vi "运维调试_五参数.vi"(11 "编号":string) -> ()   [LabVIEW 2022 SP3, in "斯坦道多参数.lvlib"]
uses:
  <vilib>/Utility/miscctls.llb/LVPointTypeDef.ctl
  <vilib>/Plasmionique/MB Master/MB_Master/MB_Master.lvclass
  <vilib>/ptbypt/NI_PtbyPt.lvlib
  <vilib>/Utility/config.llb/NI_LVConfig.lvlib
  <userlib>/_OpenG.lib/variantconfig/variantconfig.llb/openg_variant_configuration_file.lvlib
panel:
  in  "Serial Config":T1={"baud rate (bps)"=9600, "stop bits"=10, "parity"=0, "flow control"=0, "timeout"=2000, "retries"=1} {"stop bits" items=["1.0"=10, "1.5"=15, "2.0"=20]; "parity" items=["None", "Odd", "Even", "Mark", "Space"]; "flow control" items=["None", "XON/XOFF", "RTS/CTS", "XON/XOFF & RTS/CTS", "DTR/DSR", "XON/XOFF & DTR/DSR"]}
  in  "探头设置":bool
  in  "量程设置":bool
  out "显示框":T2={"显示控件"={"标题背景颜色"=3381759, "监测值背景颜色"=16777226, "监测参数"="", "状态1"="", "状态2"="", "数据标识"=""}, "显示控件 2"={"标题背景颜色"=3381759, "监测值背景颜色"=16777226, "监测参数"="", "状态1"="", "状态2"="", "数据标识"=""}, "显示控件 3"={"标题背景颜色"=3381759, "监测值背景颜色"=16777226, "监测参数"="", "状态1"="", "状态2"="", "数据标识"=""}, "显示控件 4"={"标题背景颜色"=3381759, "监测值背景颜色"=16777226, "监测参数"="", "状态1"="", "状态2"="", "数据标识"=""}, "显示控件 5"={"标题背景颜色"=3381759, "监测值背景颜色"=16777226, "监测参数"="", "状态1"="", "状态2"="", "数据标识"=""}, "显示控件 6"={"标题背景颜色"=3381759, "监测值背景颜色"=16777226, "监测参数"="", "状态1"="", "状态2"="", "数据标识"=""}, "显示控件 7"={"标题背景颜色"=3381759, "监测值背景颜色"=16777226, "监测参数"="", "状态1"="", "状态2"="", "数据标识"=""}, "显示控件 8"={"标题背景颜色"=3381759, "监测值背景颜色"=16777226, "监测参数"="", "状态1"="", "状态2"="", "数据标识"=""}, "显示控件 9"={"标题背景颜色"=3381759, "监测值背景颜色"=16777226, "监测参数"="", "状态1"="", "状态2"="", "数据标识"=""}, "显示控件 10"={"标题背景颜色"=3381759, "监测值背景颜色"=16777226, "监测参数"="", "状态1"="", "状态2"="", "数据标识"=""}}
  in  "传感器系列号":bool
  in  "水样保存组数":dbl caption="水样保存组数:"
  in  "水样稳定时间":dbl caption="水样稳定时间:"
  out "模块版本号":string
  out "权限等级":string
  in  "打开modbus":bool
  out "选项卡控件":enum32{"选项卡 1", "选项卡 2"}(tab)
  in  "VISA资源名称":refnum<visa-resource-name> caption="串口"
  in  "IP":string="localhost" caption="IP:"
  in  "Port":u16=502 caption="Port:"
  in  "自动断线重连":bool=TRUE
  in  "连接方式":u16(ring) items=["Modbus RTU", "Modbus TCP"]
  in  "密码锁":bool
  in  "设置页返回":bool
  in  "周期设置":bool
  out "当前串口":string
  out "运行状态":enum16{"空闲", "水样测试", "标样核查"}(ring)
  in  "停止":bool
  in  "标样核查":bool
  in  "水样测试":bool
  in  "设置":bool
  in  "探头校正返回":bool
  in  "探头校正":bool
  # "请设置仪器连接方式"
  # "组"
  # "min"
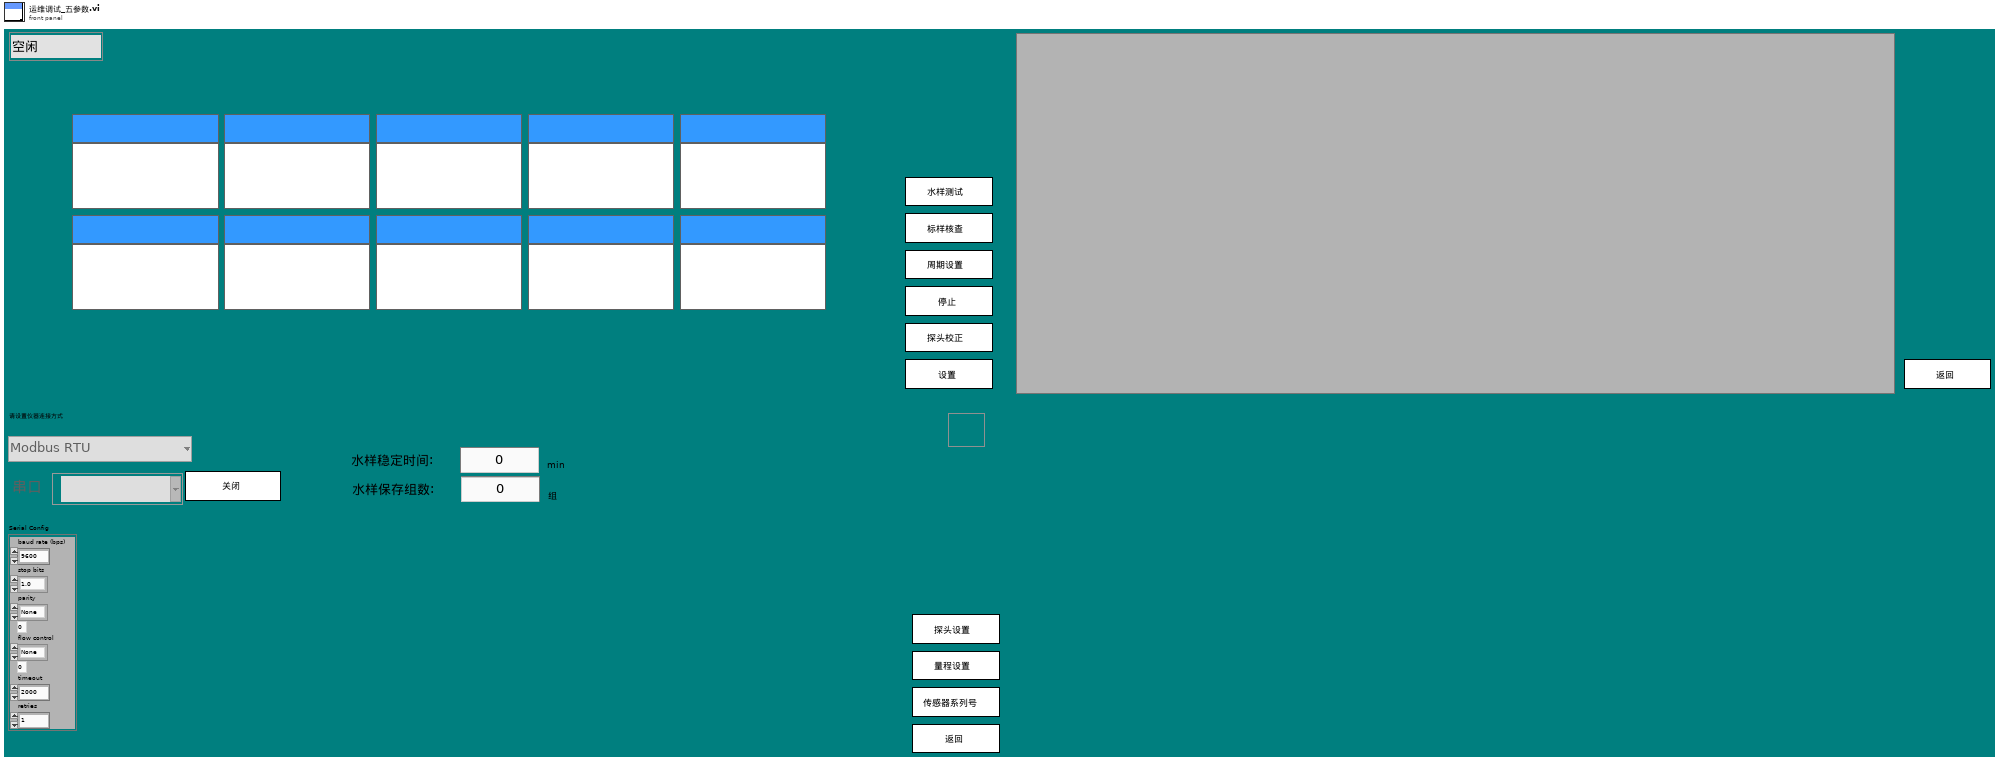
[diagram p1: front panel]
types:
  T1 = cluster{"baud rate (bps)":u32, "stop bits":u16, "parity":u16, "flow control":u16, "timeout":u32, "retries":i32}
  T2 = typedef "斯坦道多参数.lvlib/多状态显示框.ctl" = cluster{"显示控件":T3, "显示控件 2":T3, "显示控件 3":T3, "显示控件 4":T3, "显示控件 5":T3, "显示控件 6":T3, "显示控件 7":T3, "显示控件 8":T3, "显示控件 9":T3, "显示控件 10":T3}
  T3 = typedef "斯坦道多参数.lvlib/显示控件.ctl" = cluster{"标题背景颜色":u32, "监测值背景颜色":u32, "监测参数":string, "状态1":string, "状态2":string, "数据标识":string}
  T4 = typedef "斯坦道多参数.lvlib/数据流类型.ctl" = cluster{"cmd":enum16{"水样测试", "标样核查", "校准状态同步", "停止"}, "data":variant}
  T5 = typedef "LVPointTypeDef.ctl" = cluster{"Horizontal":i16, "Vertical":i16}
  T6 = enum8{"Enabled", "Disabled", "Disabled and Grayed Out"}
  T7 = cluster{"标签":string, "检测值1":cluster{"检测值":dbl, "单位":string, "启用":bool}, "检测值2":cluster{"检测值":dbl, "单位":string, "启用":bool}, "数据标识":string}[]
  T8 = cluster{"标签":string, "检测值1":cluster{"检测值":dbl, "单位":string, "启用":bool}, "检测值2":cluster{"检测值":dbl, "单位":string, "启用":bool}, "数据标识":string}
  T9 = cluster{"CH":u16, "监测值":dbl, "信号值":sgl, "数据标识":string}
  T10 = cluster{"温度测量值":sgl, "测量值":sgl, "温度偏移修正值":sgl, "信号值":sgl, "数据标识":string}
  T11 = cluster{"温度测量值":sgl, "DO%":sgl, "DOmg/L":sgl, "温度偏移修正值":sgl, "数据标识mg/L":string, "数据标识%":string}
  T12 = cluster{"周期设置类型":enum16{"定点启动", "间隔启动"}, "定时功能启用":bool, "定时间隔":u32, "24H周期设置":bool[], "延迟启动时间":u32}
  T13 = typedef "LVDateTimeRec.ctl" = cluster{"秒数的小数部分":dbl, "秒":i32, "分":i32, "时":i32, "日":i32, "月":i32, "年":i32, "天数（周）":i32, "天数（年）":i32, "DST":i32}
  T14 = cluster{"运行模式":enum16{"维护模式", "常规模式", "应急模式", "质控模式"}, "24H周期设置":bool[]}
  T15 = cluster{"Major":u16, "Minor":u16, "Fix":u16, "Build":u16}
  T16 = typedef "NI_LVConfig.lvlib/Config Data RefNum.ctl" = refnum<k1>
  T17 = enum32{"Bad", "Idle", "Run top level", "Running"}
  T18 = cluster{"ph":bool, "DO":bool, "Cond":bool, "Turb":bool, "叶绿素a":bool, "藻密度":bool, "ORP":bool, "cod":bool, "DO2":bool, "氯化物":bool, "氨氮":bool, "水中油":bool, "悬浮物":bool, "余氯":bool}
  T19 = cluster{"水温 (℃)":cluster{"量程下限":dbl, "量程上限":dbl}, "DO (mg/L)":cluster{"量程下限":dbl, "量程上限":dbl}, "DO (%)":cluster{"量程下限":dbl, "量程上限":dbl}, "pH":cluster{"量程下限":dbl, "量程上限":dbl}, "电导率 (μS/cm)":cluster{"量程下限":dbl, "量程上限":dbl}, "盐度":cluster{"量程下限":dbl, "量程上限":dbl}, "浊度 (NTU)":cluster{"量程下限":dbl, "量程上限":dbl}, "叶绿素a (μg/L)":cluster{"量程下限":dbl, "量程上限":dbl}, "藻密度 (cells/mL)":cluster{"量程下限":dbl, "量程上限":dbl}, "ORP (mV)":cluster{"量程下限":dbl, "量程上限":dbl}, "氯化物（mg/L）":cluster{"量程下限":dbl, "量程上限":dbl}, "COD":cluster{"量程下限":dbl, "量程上限":dbl}, "氨氮":cluster{"量程下限":dbl, "量程上限":dbl}, "水中油":cluster{"量程下限":dbl, "量程上限":dbl}, "悬浮物":cluster{"量程下限":dbl, "量程上限":dbl}, "余氯":cluster{"量程下限":dbl, "量程上限":dbl}}
  T20 = cluster{"周期设置类型":enum16{"定点启动", "间隔启动"}, "定时功能启用":bool, "定时间隔":u32, "24H周期设置":bool[], "延时启动时间":u32}
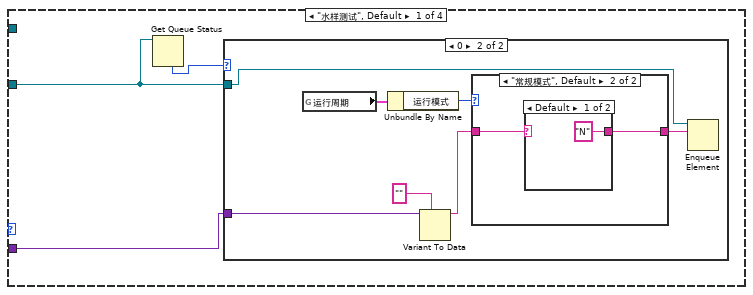
[diagram p2: hidden frame]
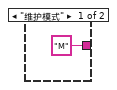
[diagram p4: hidden frame]
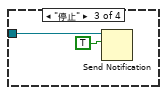
[diagram p7: hidden frame]
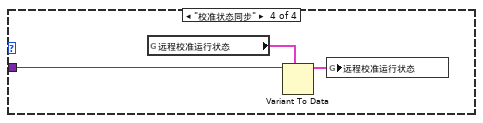
[diagram p8: hidden frame]
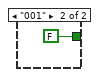
[diagram p9: hidden frame]
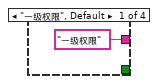
[diagram p17: hidden frame]
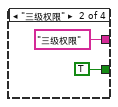
[diagram p18: hidden frame]
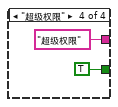
[diagram p19: hidden frame]
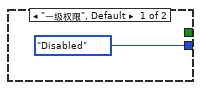
[diagram p20: hidden frame]
diagram:
  n1 = control-ref of="本VI"() -> (w22:refnum<vi>)
  n2 = while {
    stop <- FALSE stop-if-true
    n3 = global read "多参数全局变量.vi" "多参数运行状态"() -> (→"运行状态":u16)
    n4 = Wait (ms)(milliseconds to wait=u32 1000 ("等待时间（毫秒）")) -> ()  [unwired: 1 out]
  }
  n5 = call "程序默认配置.vi"() -> ()  [unwired: 11 in, 1 out]
  n6 = while {
    stop <- FALSE stop-if-true
    # "配置"
    n7 = global read "断电保存变量.vi" "Port"() -> (w55:u16)
    n8 = global read "断电保存变量.vi" "IP"() -> (w56:string)
    n9 = global read "断电保存变量.vi" "连接方式"() -> (w49:u16)
    "选项卡控件" <- w49
    n10 = global read "多参数全局变量.vi" "MB session in"() -> (w64:refnum<class "MB_Master.lvclass">)
    n11 = Wait (ms)(milliseconds to wait=u32 500 ("等待时间（毫秒）")) -> ()  [unwired: 1 out]
    n12 = global read "断电保存变量.vi" "VISA资源名称"() -> (w52:refnum<visa-resource-name>)
    n13 = global read "断电保存变量.vi" "Serial Config"() -> (w40:T1)
    n14 = global read "断电保存变量.vi" "水样稳定时间"() -> (w43:dbl)
    n15 = global read "断电保存变量.vi" "水样测试组数"() -> (w41:dbl)
    n16 = global read "断电保存变量.vi" "自动断线重连"() -> (w44:bool)
    n17 = local write "IP"(w56) -> ()
    n18 = local write "Port"(w55) -> ()
    n19 = global read "断电保存变量.vi" "连接方式"() -> (w53:u16)
    n20 = local write "连接方式"(w49) -> ()
    n21 = local write "Serial Config"(w40) -> ()
    n22 = local write "水样稳定时间"(w43) -> ()
    n23 = global read "多参数全局变量.vi" "MB session in"() -> (w67:refnum<class "MB_Master.lvclass">)
    n24 = local write "水样保存组数"(w41) -> ()
    n25 = local write "自动断线重连"(w44) -> ()
    n26 = local write "VISA资源名称"(w52) -> ()
    n27 = case shown="1" w53 {
      tunnel: w52 -> [w69 _]
      tunnel: [w69 w70] -> w51
      frame 0, Default {
      }
      frame 1 {
        n28 = global read "断电保存变量.vi" "Port"() -> (w71:u16)
        n29 = global read "断电保存变量.vi" "IP"() -> (w73:string)
        n30 = Format Into String(format string=":%d" ("格式字符串"), initial string=w73, w71) -> (resulting string=w70:string)  [unwired: 1 in, 1 out]
      }
    }
    "当前串口" <- w51
    n31 = property class="MB_Master"(reference=w64) -> ("Properties:Session Valid"=w48:bool)  [unwired: 1 in, 2 out]
    n32 = local read "密码锁"() -> (w60:bool)
    n33 = property class="MB_Master"(reference=w67) -> ("Properties:Session Valid"=w66:bool)  [unwired: 1 in, 2 out]
    n34 = Select(t=T6."Enabled" ("f"), s=w60, f=T6."Disabled") -> (s? t:f=w58:T6)
    n35 = Not(x=w48) -> (.not. x?=w50:bool)
    n36 = Select(t="关闭" ("布尔文本.文本"), s=w48, f="打开" ("布尔文本.文本")) -> (s? t:f=w61:string)
    n37 = Select(t=u32 16777216, s=w48, f=u32 16722483) -> (s? t:f=w45:u32)
    n38 = property on="当前串口" class="Str"("Blinking"=w50, "Text.BG Color"=w45) -> ()  [unwired: 2 in, 2 out]
    n39 = Select(t=T6."Disabled and Grayed Out" ("禁用"), s=w66, f=w58) -> (s? t:f=w54:T6)
    n40 = property on="IP" class="Str"("DisabledEnum"=w54) -> ()  [unwired: 2 in, 2 out]
    n41 = property on="Port" class="DigNum (strict)"("DisabledEnum"=w54) -> ()  [unwired: 2 in, 2 out]
    n42 = property on="VISA资源名称" class="VISAName"("DisabledEnum"=w54) -> ()  [unwired: 2 in, 2 out]
    n43 = property on="连接方式" class="Ring (strict)"("DisabledEnum"=w54) -> ()  [unwired: 2 in, 2 out]
    n44 = property on="打开modbus" class="Bool"("BoolText.Text"=w61) -> ()  [unwired: 2 in, 2 out]
  }
  n45 = call "taskqueue ref.vi"() -> ("队列输出"=w5:refnum<queue>)  [unwired: 10 in, 1 out]
  n46 = while {
    stop <- FALSE stop-if-true
    # "显示处理"
    n47 = global read "断电保存变量.vi" "Temp"() -> (w121:bool)
    n48 = Wait (ms)(milliseconds to wait=u32 1000 ("等待时间（毫秒）")) -> ()  [unwired: 1 out]
    n49 = case shown="True" w121 {
      tunnel: [w401 w413] -> w118
      tunnel: T7 [] ("数组") -> [w401 w414]
      tunnel: [T6."Disabled and Grayed Out" ("禁用") T6."Enabled" ("禁用")] -> _
      tunnel: string[] [] -> [w399 w404]
      tunnel: [w399 w403] -> w104
      frame False {
      }
      frame True {
        n50 = global read "多参数全局变量.vi" "水温显示"() -> (w411:T9)
        n51 = Insert Into Array(array=w404, new element="水温" ("新元素/子数组")) -> (w403:string[])  [unwired: 1 in]
        n52 = Unbundle By Name(w411) -> ("CH"=w410:u16, "监测值"=w408:dbl, "数据标识"=w407:string)
        n53 = case shown="4" w410 {
          tunnel: ["水温 Temp (pH)" ("监测参数1") "水温 Temp (DO)" ("监测参数1") "水温 Temp (浊度)" ("监测参数1") "水温 Temp (电导率)" ("监测参数1") "水温 Temp (叶绿素a)" ("监测参数1") "水温 Temp (藻密度)" ("监测参数1")] -> w416
          frame 0, Default {
          }
          frame 1 {
          }
          frame 2 {
          }
          frame 3 {
          }
          frame 4 {
          }
          frame 5 {
          }
        }
        n54 = Bundle By Name(cluster=T8 {"标签"="", "检测值1"={"检测值"=0.0, "单位"="", "启用"=FALSE}, "检测值2"={"检测值"=0.0, "单位"="", "启用"=FALSE}, "数据标识"=""} ("多参数状态显示"), "标签"=w416, "检测值1.检测值"=w408, "检测值1.单位"="℃", "检测值1.启用"=TRUE, "数据标识"=w407) -> (w415:T8)
        n55 = Insert Into Array(array=w414, new element=w415) -> (w413:T7)  [unwired: 1 in]
      }
    }
    n56 = global read "断电保存变量.vi" "pH"() -> (w119:bool)
    n57 = case shown="True" w119 {
      tunnel: [w382 w397] -> w116
      tunnel: w118 -> [w382 w398]
      tunnel: [T6."Disabled and Grayed Out" ("禁用") T6."Enabled" ("禁用")] -> _
      tunnel: w104 -> [w380 w385]
      tunnel: [w380 w384] -> w103
      frame False {
      }
      frame True {
        (unwired) "%.2f(%.2f mV)" ("格式字符串")
        n58 = global read "多参数全局变量.vi" "ph显示"() -> (w395:T10)
        n59 = Insert Into Array(array=w385, new element="pH" ("新元素/子数组")) -> (w384:string[])  [unwired: 1 in]
        n60 = Unbundle By Name(w395) -> ("测量值"=w392:sgl, "信号值"=w390:sgl, "数据标识"=w388:string)
        n61 = Bundle By Name(cluster=T8 {"标签"="", "检测值1"={"检测值"=0.0, "单位"="", "启用"=FALSE}, "检测值2"={"检测值"=0.0, "单位"="", "启用"=FALSE}, "数据标识"=""} ("多参数状态显示"), "标签"="酸碱度 pH" ("监测参数2"), "检测值1.检测值"=w392, "检测值1.启用"=TRUE, "检测值2.检测值"=w390, "检测值2.单位"="mV", "检测值2.启用"=TRUE, "数据标识"=w388) -> (w386:T8)
        n62 = Insert Into Array(array=w398, new element=w386) -> (w397:T7)  [unwired: 1 in]
      }
    }
    n63 = global read "断电保存变量.vi" "DO"() -> (w117:bool)
    n64 = case shown="True" w117 {
      tunnel: [w362 w378] -> w97
      tunnel: w116 -> [w362 w379]
      tunnel: [T6."Disabled and Grayed Out" ("禁用") T6."Enabled" ("禁用")] -> _
      tunnel: w103 -> [w360 w365]
      tunnel: [w360 w364] -> w96
      frame False {
      }
      frame True {
        n65 = global read "多参数全局变量.vi" "DO显示"() -> (w376:T11)
        n66 = Insert Into Array(array=w365, new element="溶解氧" ("新元素/子数组")) -> (w364:string[])  [unwired: 1 in]
        n67 = Unbundle By Name(w376) -> ("DOmg/L"=w373:sgl, "DO%"=w371:sgl, "数据标识mg/L"=w370:string)
        n68 = Bundle By Name(cluster=T8 {"标签"="", "检测值1"={"检测值"=0.0, "单位"="", "启用"=FALSE}, "检测值2"={"检测值"=0.0, "单位"="", "启用"=FALSE}, "数据标识"=""} ("多参数状态显示"), "标签"="溶解氧 DO" ("监测参数2"), "检测值1.检测值"=w373, "检测值1.单位"="mg/L", "检测值1.启用"=TRUE, "检测值2.检测值"=w371, "检测值2.单位"="%", "检测值2.启用"=TRUE, "数据标识"=w370) -> (w366:T8)
        n69 = Insert Into Array(array=w379, new element=w366) -> (w378:T7)  [unwired: 1 in]
      }
    }
    n70 = global read "断电保存变量.vi" "DO 2"() -> (w98:bool)
    n71 = case shown="True" w98 {
      tunnel: [w221 w237] -> w95
      tunnel: w97 -> [w221 w238]
      tunnel: [T6."Disabled and Grayed Out" ("禁用") T6."Enabled" ("禁用")] -> _
      tunnel: w96 -> [w219 w224]
      tunnel: [w219 w223] -> w94
      frame False {
      }
      frame True {
        n72 = global read "多参数全局变量.vi" "DO2显示"() -> (w235:T11)
        n73 = Insert Into Array(array=w224, new element="溶解氧" ("新元素/子数组")) -> (w223:string[])  [unwired: 1 in]
        n74 = Unbundle By Name(w235) -> ("DOmg/L"=w232:sgl, "DO%"=w230:sgl, "数据标识mg/L"=w229:string)
        n75 = Bundle By Name(cluster=T8 {"标签"="", "检测值1"={"检测值"=0.0, "单位"="", "启用"=FALSE}, "检测值2"={"检测值"=0.0, "单位"="", "启用"=FALSE}, "数据标识"=""} ("多参数状态显示"), "标签"="溶解氧 DO2" ("监测参数2"), "检测值1.检测值"=w232, "检测值1.单位"="mg/L", "检测值1.启用"=TRUE, "检测值2.检测值"=w230, "检测值2.单位"="%", "检测值2.启用"=TRUE, "数据标识"=w229) -> (w225:T8)
        n76 = Insert Into Array(array=w238, new element=w225) -> (w237:T7)  [unwired: 1 in]
      }
    }
    n77 = global read "断电保存变量.vi" "Cond"() -> (w115:bool)
    n78 = case shown="True" w115 {
      tunnel: w95 -> [w334 w359]
      tunnel: [w334 w355] -> w108
      tunnel: [T6."Disabled and Grayed Out" ("禁用") T6."Enabled" ("禁用")] -> _
      tunnel: w94 -> [w332 w339]
      tunnel: [w332 w338] -> w102
      frame False {
      }
      frame True {
        n79 = global read "多参数全局变量.vi" "spcond显示"() -> (w357:T10)
        n80 = Insert Into Array(array=w339, new element="电导率" ("新元素/子数组")) -> (w338:string[])  [unwired: 1 in]
        n81 = global read "多参数全局变量.vi" "盐度显示"() -> (w354:T10)
        n82 = Unbundle By Name(w357) -> ("测量值"=w348:sgl, "数据标识"=w346:string, "信号值"=w336:sgl)
        n83 = Unbundle By Name(w354) -> ("测量值"=w343:sgl, "数据标识"=w342:string)
        n84 = Bundle By Name(cluster=T8 {"标签"="", "检测值1"={"检测值"=0.0, "单位"="", "启用"=FALSE}, "检测值2"={"检测值"=0.0, "单位"="", "启用"=FALSE}, "数据标识"=""} ("多参数状态显示"), "标签"="电导率 Cond" ("监测参数2"), "检测值1.检测值"=w348, "检测值1.单位"="μS/cm", "检测值1.启用"=TRUE, "数据标识"=w346, "检测值2.检测值"=w336, "检测值2.启用"=TRUE) -> (w345:T8)
        n85 = Bundle By Name(cluster=T8 {"标签"="", "检测值1"={"检测值"=0.0, "单位"="", "启用"=FALSE}, "检测值2"={"检测值"=0.0, "单位"="", "启用"=FALSE}, "数据标识"=""} ("多参数状态显示"), "标签"="盐度 Sal" ("监测参数2"), "检测值1.检测值"=w343, "检测值1.单位"="ppt" ("检测值2.单位"), "检测值1.启用"=TRUE, "数据标识"=w342) -> (w340:T8)
        n86 = Insert Into Array(array=w359, new element=w345) -> (w356:T7)  [unwired: 1 in]
        n87 = Insert Into Array(array=w356, new element=w340) -> (w355:T7)  [unwired: 1 in]
      }
    }
    n88 = global read "断电保存变量.vi" "orp"() -> (w110:bool)
    n89 = case shown="True" w110 {
      tunnel: w108 -> [w260 w274]
      tunnel: [w260 w273] -> w109
      tunnel: [T6."Disabled and Grayed Out" ("禁用") T6."Enabled" ("禁用")] -> _
      tunnel: w102 -> [w258 w263]
      tunnel: [w258 w262] -> w101
      frame False {
      }
      frame True {
        n90 = global read "多参数全局变量.vi" "ORP显示"() -> (w271:T10)
        n91 = Insert Into Array(array=w263, new element="ORP" ("新元素/子数组")) -> (w262:string[])  [unwired: 1 in]
        n92 = Unbundle By Name(w271) -> ("测量值"=w266:sgl, "数据标识"=w265:string)
        n93 = Bundle By Name(cluster=T8 {"标签"="", "检测值1"={"检测值"=0.0, "单位"="", "启用"=FALSE}, "检测值2"={"检测值"=0.0, "单位"="", "启用"=FALSE}, "数据标识"=""} ("多参数状态显示"), "标签"="ORP" ("监测参数2"), "检测值1.检测值"=w266, "检测值1.单位"="mV", "检测值1.启用"=TRUE, "数据标识"=w265) -> (w264:T8)
        n94 = Insert Into Array(array=w274, new element=w264) -> (w273:T7)  [unwired: 1 in]
      }
    }
    n95 = global read "断电保存变量.vi" "Turb"() -> (w114:bool)
    n96 = case shown="True" w114 {
      tunnel: w109 -> [w315 w331]
      tunnel: [w315 w330] -> w81
      tunnel: [T6."Disabled and Grayed Out" ("禁用") T6."Enabled" ("禁用")] -> _
      tunnel: w101 -> [w313 w320]
      tunnel: [w313 w319] -> w83
      frame False {
      }
      frame True {
        n97 = global read "多参数全局变量.vi" "浊度显示"() -> (w328:T10)
        n98 = Insert Into Array(array=w320, new element="浊度" ("新元素/子数组")) -> (w319:string[])  [unwired: 1 in]
        n99 = Unbundle By Name(w328) -> ("测量值"=w323:sgl, "数据标识"=w322:string, "信号值"=w317:sgl)
        n100 = Bundle By Name(cluster=T8 {"标签"="", "检测值1"={"检测值"=0.0, "单位"="", "启用"=FALSE}, "检测值2"={"检测值"=0.0, "单位"="", "启用"=FALSE}, "数据标识"=""} ("多参数状态显示"), "标签"="浊度 Turb" ("监测参数2"), "检测值1.检测值"=w323, "检测值1.单位"="NTU", "检测值1.启用"=TRUE, "数据标识"=w322, "检测值2.检测值"=w317, "检测值2.启用"=TRUE) -> (w321:T8)
        n101 = Insert Into Array(array=w331, new element=w321) -> (w330:T7)  [unwired: 1 in]
      }
    }
    n102 = global read "断电保存变量.vi" "SS"() -> (w79:bool)
    n103 = case shown="True" w79 {
      tunnel: w81 -> [w145 w161]
      tunnel: [w145 w160] -> w80
      tunnel: [T6."Disabled and Grayed Out" ("禁用") T6."Enabled" ("禁用")] -> _
      tunnel: w83 -> [w143 w150]
      tunnel: [w143 w149] -> w82
      frame False {
      }
      frame True {
        n104 = global read "多参数全局变量.vi" "悬浮物显示"() -> (w158:T10)
        n105 = Insert Into Array(array=w150, new element="悬浮物" ("新元素/子数组")) -> (w149:string[])  [unwired: 1 in]
        n106 = Unbundle By Name(w158) -> ("测量值"=w153:sgl, "数据标识"=w152:string, "信号值"=w147:sgl)
        n107 = Bundle By Name(cluster=T8 {"标签"="", "检测值1"={"检测值"=0.0, "单位"="", "启用"=FALSE}, "检测值2"={"检测值"=0.0, "单位"="", "启用"=FALSE}, "数据标识"=""} ("多参数状态显示"), "标签"="悬浮物 SS" ("监测参数2"), "检测值1.检测值"=w153, "检测值1.单位"="mg/L", "检测值1.启用"=TRUE, "数据标识"=w152, "检测值2.检测值"=w147, "检测值2.启用"=TRUE) -> (w151:T8)
        n108 = Insert Into Array(array=w161, new element=w151) -> (w160:T7)  [unwired: 1 in]
      }
    }
    n109 = global read "断电保存变量.vi" "叶绿素a启用"() -> (w113:bool)
    n110 = case shown="True" w113 {
      tunnel: w80 -> [w296 w312]
      tunnel: [w296 w311] -> w111
      tunnel: [T6."Disabled and Grayed Out" ("禁用") T6."Enabled" ("禁用")] -> _
      tunnel: w82 -> [w294 w305]
      tunnel: [w294 w304] -> w100
      frame False {
      }
      frame True {
        n111 = global read "多参数全局变量.vi" "叶绿素a显示"() -> (w299:T10)
        n112 = Insert Into Array(array=w305, new element="叶绿素a" ("新元素/子数组")) -> (w304:string[])  [unwired: 1 in]
        n113 = Unbundle By Name(w299) -> ("信号值"=w298:sgl)
        n114 = call "叶绿素a单位换算.vi"("叶绿素a显示"=w299) -> ("数据标识"=w300:string, "检测值1.单位"=w302:string, "测量值"=w301:sgl)  [unwired: 8 in]
        n115 = Bundle By Name(cluster=T8 {"标签"="", "检测值1"={"检测值"=0.0, "单位"="", "启用"=FALSE}, "检测值2"={"检测值"=0.0, "单位"="", "启用"=FALSE}, "数据标识"=""} ("多参数状态显示"), "标签"="叶绿素a Chla" ("监测参数2"), "检测值1.检测值"=w301, "检测值1.单位"=w302, "检测值1.启用"=TRUE, "数据标识"=w300, "检测值2.检测值"=w298, "检测值2.启用"=TRUE) -> (w306:T8)
        n116 = Insert Into Array(array=w312, new element=w306) -> (w311:T7)  [unwired: 1 in]
      }
    }
    n117 = global read "断电保存变量.vi" "藻密度"() -> (w112:bool)
    n118 = case shown="True" w112 {
      tunnel: w111 -> [w277 w293]
      tunnel: [w277 w292] -> w107
      tunnel: [T6."Disabled and Grayed Out" ("禁用") T6."Enabled" ("禁用")] -> _
      tunnel: w100 -> [w275 w286]
      tunnel: [w275 w285] -> w99
      frame False {
      }
      frame True {
        n119 = global read "多参数全局变量.vi" "藻密度显示"() -> (w280:T10)
        n120 = Insert Into Array(array=w286, new element="藻密度" ("新元素/子数组")) -> (w285:string[])  [unwired: 1 in]
        n121 = Unbundle By Name(w280) -> ("信号值"=w279:sgl)
        n122 = call "藻密度单位换算.vi"("藻密度显示"=w280) -> ("数据标识"=w282:string, "检测值1.单位"=w281:string, "测量值"=w283:sgl)  [unwired: 8 in]
        n123 = Bundle By Name(cluster=T8 {"标签"="", "检测值1"={"检测值"=0.0, "单位"="", "启用"=FALSE}, "检测值2"={"检测值"=0.0, "单位"="", "启用"=FALSE}, "数据标识"=""} ("多参数状态显示"), "标签"="藻密度 Algal" ("监测参数2"), "检测值1.检测值"=w283, "检测值1.单位"=w281, "检测值1.启用"=TRUE, "数据标识"=w282, "检测值2.检测值"=w279, "检测值2.启用"=TRUE) -> (w287:T8)
        n124 = Insert Into Array(array=w293, new element=w287) -> (w292:T7)  [unwired: 1 in]
      }
    }
    n125 = global read "断电保存变量.vi" "COD"() -> (w106:bool)
    n126 = case shown="True" w106 {
      tunnel: w107 -> [w241 w257]
      tunnel: [w241 w256] -> w90
      tunnel: [T6."Disabled and Grayed Out" ("禁用") T6."Enabled" ("禁用")] -> _
      tunnel: w99 -> [w239 w246]
      tunnel: [w239 w245] -> w91
      frame False {
      }
      frame True {
        n127 = global read "多参数全局变量.vi" "COD显示"() -> (w254:T10)
        n128 = Insert Into Array(array=w246, new element="COD" ("新元素/子数组")) -> (w245:string[])  [unwired: 1 in]
        n129 = Unbundle By Name(w254) -> ("测量值"=w249:sgl, "数据标识"=w248:string, "信号值"=w243:sgl)
        n130 = Bundle By Name(cluster=T8 {"标签"="", "检测值1"={"检测值"=0.0, "单位"="", "启用"=FALSE}, "检测值2"={"检测值"=0.0, "单位"="", "启用"=FALSE}, "数据标识"=""} ("多参数状态显示"), "标签"="COD" ("监测参数2"), "检测值1.检测值"=w249, "检测值1.单位"="mg/L", "检测值1.启用"=TRUE, "数据标识"=w248, "检测值2.检测值"=w243, "检测值2.启用"=TRUE) -> (w247:T8)
        n131 = Insert Into Array(array=w257, new element=w247) -> (w256:T7)  [unwired: 1 in]
      }
    }
    n132 = global read "断电保存变量.vi" "氯化物"() -> (w92:bool)
    n133 = case shown="True" w92 {
      tunnel: w90 -> [w202 w218]
      tunnel: [w202 w217] -> w88
      tunnel: [T6."Disabled and Grayed Out" ("禁用") T6."Enabled" ("禁用")] -> _
      tunnel: w91 -> [w200 w207]
      tunnel: [w200 w206] -> w89
      frame False {
      }
      frame True {
        n134 = global read "多参数全局变量.vi" "氯化物显示"() -> (w215:T10)
        n135 = Insert Into Array(array=w207, new element="氯化物" ("新元素/子数组")) -> (w206:string[])  [unwired: 1 in]
        n136 = Unbundle By Name(w215) -> ("测量值"=w210:sgl, "数据标识"=w209:string, "信号值"=w204:sgl)
        n137 = Bundle By Name(cluster=T8 {"标签"="", "检测值1"={"检测值"=0.0, "单位"="", "启用"=FALSE}, "检测值2"={"检测值"=0.0, "单位"="", "启用"=FALSE}, "数据标识"=""} ("多参数状态显示"), "标签"="氯化物" ("监测参数2"), "检测值1.检测值"=w210, "检测值1.单位"="mg/L", "检测值1.启用"=TRUE, "数据标识"=w209, "检测值2.检测值"=w204, "检测值2.启用"=TRUE) -> (w208:T8)
        n138 = Insert Into Array(array=w218, new element=w208) -> (w217:T7)  [unwired: 1 in]
      }
    }
    n139 = global read "断电保存变量.vi" "氨氮"() -> (w87:bool)
    n140 = case shown="True" w87 {
      tunnel: w88 -> [w183 w199]
      tunnel: [w183 w198] -> w85
      tunnel: [T6."Disabled and Grayed Out" ("禁用") T6."Enabled" ("禁用")] -> _
      tunnel: w89 -> [w181 w188]
      tunnel: [w181 w187] -> w86
      frame False {
      }
      frame True {
        n141 = global read "多参数全局变量.vi" "氨氮显示"() -> (w196:T10)
        n142 = Insert Into Array(array=w188, new element="氨氮" ("新元素/子数组")) -> (w187:string[])  [unwired: 1 in]
        n143 = Unbundle By Name(w196) -> ("测量值"=w191:sgl, "数据标识"=w190:string, "信号值"=w185:sgl)
        n144 = Bundle By Name(cluster=T8 {"标签"="", "检测值1"={"检测值"=0.0, "单位"="", "启用"=FALSE}, "检测值2"={"检测值"=0.0, "单位"="", "启用"=FALSE}, "数据标识"=""} ("多参数状态显示"), "标签"="氨氮" ("监测参数2"), "检测值1.检测值"=w191, "检测值1.单位"="mg/L", "检测值1.启用"=TRUE, "数据标识"=w190, "检测值2.检测值"=w185, "检测值2.启用"=TRUE) -> (w189:T8)
        n145 = Insert Into Array(array=w199, new element=w189) -> (w198:T7)  [unwired: 1 in]
      }
    }
    n146 = global read "断电保存变量.vi" "水中油"() -> (w84:bool)
    n147 = case shown="True" w84 {
      tunnel: w85 -> [w164 w180]
      tunnel: [w164 w179] -> w76
      tunnel: [T6."Disabled and Grayed Out" ("禁用") T6."Enabled" ("禁用")] -> _
      tunnel: w86 -> [w162 w169]
      tunnel: [w162 w168] -> w77
      frame False {
      }
      frame True {
        n148 = global read "多参数全局变量.vi" "水中油显示"() -> (w177:T10)
        n149 = Insert Into Array(array=w169, new element="水中油" ("新元素/子数组")) -> (w168:string[])  [unwired: 1 in]
        n150 = Unbundle By Name(w177) -> ("测量值"=w172:sgl, "数据标识"=w171:string, "信号值"=w166:sgl)
        n151 = Bundle By Name(cluster=T8 {"标签"="", "检测值1"={"检测值"=0.0, "单位"="", "启用"=FALSE}, "检测值2"={"检测值"=0.0, "单位"="", "启用"=FALSE}, "数据标识"=""} ("多参数状态显示"), "标签"="水中油" ("监测参数2"), "检测值1.检测值"=w172, "检测值1.单位"="mg/L", "检测值1.启用"=TRUE, "数据标识"=w171, "检测值2.检测值"=w166, "检测值2.启用"=TRUE) -> (w170:T8)
        n152 = Insert Into Array(array=w180, new element=w170) -> (w179:T7)  [unwired: 1 in]
      }
    }
    n153 = global read "断电保存变量.vi" "余氯"() -> (w78:bool)
    n154 = case shown="True" w78 {
      tunnel: w76 -> [w126 w142]
      tunnel: [w126 w141] -> w75
      tunnel: [T6."Disabled and Grayed Out" ("禁用") T6."Enabled" ("禁用")] -> _
      tunnel: w77 -> [w124 w131]
      tunnel: [w124 w130] -> w74
      frame False {
      }
      frame True {
        n155 = global read "多参数全局变量.vi" "余氯显示"() -> (w139:T10)
        n156 = Insert Into Array(array=w131, new element="余氯" ("新元素/子数组")) -> (w130:string[])  [unwired: 1 in]
        n157 = Unbundle By Name(w139) -> ("测量值"=w134:sgl, "数据标识"=w133:string, "信号值"=w128:sgl)
        n158 = Bundle By Name(cluster=T8 {"标签"="", "检测值1"={"检测值"=0.0, "单位"="", "启用"=FALSE}, "检测值2"={"检测值"=0.0, "单位"="", "启用"=FALSE}, "数据标识"=""} ("多参数状态显示"), "标签"="余氯" ("监测参数2"), "检测值1.检测值"=w134, "检测值1.单位"="mg/L", "检测值1.启用"=TRUE, "数据标识"=w133, "检测值2.检测值"=w128, "检测值2.启用"=TRUE) -> (w132:T8)
        n159 = Insert Into Array(array=w142, new element=w132) -> (w141:T7)  [unwired: 1 in]
      }
    }
    n160 = control-ref of="显示框"() -> (w93:refnum<vi>)
    n161 = global write "多参数全局变量.vi" "启动参数名称"(w74) -> ()
    n162 = call "显示转换.vi"("显示控件"=w93, "数组输入"=w75) -> ()  [unwired: 10 in]
  }
  n163 = call "task.vi"() -> ()  [unwired: 12 in]
  n164 = while {
    shift-right: [w433] -> _
    shift-left: u32 0 ("等待时间（毫秒）") -> [w434]
    stop <- FALSE stop-if-true
    # "密码权限"
    n165 = global read "多参数全局变量.vi" "权限"() -> (w425:enum16{"一级权限", "二级权限", "三级权限", "超级权限"})
    n166 = global read "多参数全局变量.vi" "权限"() -> (w426:enum16{"一级权限", "二级权限", "三级权限", "超级权限"})
    n167 = local read "连接方式"() -> (w430:u16)
    n168 = local read "密码锁"() -> (w435:bool)
    n169 = Wait (ms)(milliseconds to wait=u32 1000 ("等待时间（毫秒）")) -> ()  [unwired: 1 out]
    n170 = case shown="\"二级权限\"..\"超级权限\"" w425 {
      tunnel: [T6."Disabled" ("禁用") T6."Enabled" ("禁用")] -> w428
      tunnel: [_ TRUE ("可见")] -> w424
      frame "一级权限", Default {
      }
      frame "二级权限".."超级权限" {
      }
    }
    n171 = case shown="\"二级权限\"" w426 {
      tunnel: ["一级权限" ("权限等级") "三级权限" ("权限等级") "二级权限" ("权限等级") "超级权限" ("权限等级")] -> w427
      tunnel: [_ TRUE FALSE TRUE] -> w423
      frame "一级权限", Default {
      }
      frame "三级权限" {
      }
      frame "二级权限" {
      }
      frame "超级权限" {
      }
    }
    "权限等级" <- w427
    n172 = case shown="1" w430 {
      tunnel: [_ TRUE ("可见")] -> w429
      frame 0, Default {
      }
      frame 1 {
      }
    }
    n173 = case shown="True" w435 {
      tunnel: w434 -> [_ w441]
      tunnel: [_ w440] -> w433
      frame False {
      }
      frame True {
        n174 = Increment(x=w441) -> (x+1=w440:u32)
      }
    }
    n175 = property on="探头设置" class="Bool"("Visible"=w423) -> ()  [unwired: 2 in, 2 out]
    n176 = property on="自动断线重连" class="Bool (strict)"("Visible"=w429) -> ()  [unwired: 2 in, 2 out]
    n177 = property on="Serial Config" class="Clust (strict)"("Visible"=w423) -> ()  [unwired: 2 in, 2 out]
    n178 = Greater Or Equal?(x=w433, y=u32 3600) -> (x >= y?=w431:bool)
    n179 = local write "密码锁"(w424) -> ()
    n180 = property on="自动断线重连" class="Bool (strict)"("DisabledEnum"=w428) -> ()  [unwired: 2 in, 2 out]
    n181 = property on="打开modbus" class="Bool"("DisabledEnum"=w428) -> ()  [unwired: 2 in, 2 out]
    n182 = case shown="True" w431 {
      frame False {
      }
      frame True {
        n183 = global write "多参数全局变量.vi" "权限"(enum16{"一级权限", "二级权限", "三级权限", "超级权限"}."一级权限" ("权限")) -> ()
      }
    }
  }
  n184 = while {
    shift-right: [w454] -> _
    shift-left: u32 0 ("等待时间（毫秒）") -> [w455]
    tunnel: w5 -> [w452]
    stop <- FALSE stop-if-true
    # "周期控制"
    n185 = global read "断电保存变量.vi" "定时控制输入"() -> (w457:T12)
    n186 = Wait (ms)(milliseconds to wait=u32 500 ("等待时间（毫秒）")) -> ()  [unwired: 1 out]
    n187 = Unbundle By Name(w457) -> ("周期设置类型"=w459:enum16{"定点启动", "间隔启动"}, "24H周期设置"=w458:bool[], "定时间隔"=w456:u32, "定时功能启用"=w453:bool)
    n188 = case shown="True" w453 {
      tunnel: w459 -> [_ w470]
      tunnel: w458 -> [_ w469]
      tunnel: w456 -> [_ w468]
      tunnel: w455 -> [_ w467]
      tunnel: [_ w466] -> w454
      tunnel: w452 -> [_ w465]
      frame False {
      }
      frame True {
        n189 = Get Date/Time In Seconds() -> (seconds since 1Jan1904=w471:timestamp)
        n190 = case shown="\"间隔启动\"" w470 {
          tunnel: w471 -> [w487 _]
          tunnel: w469 -> [w484 _]
          tunnel: [w478 w495] -> w464
          tunnel: w468 -> [_ w494]
          tunnel: w467 -> [_ w496]
          tunnel: [_ w490] -> w466
          frame "定点启动", Default {
            n191 = Seconds To Date/Time(time stamp (now)=w487) -> (date time rec=w486:T13)  [unwired: 1 in]
            n192 = Unbundle By Name(w486) -> ("时"=w485:i32, "分"=w483:i32, "秒"=w482:i32)
            n193 = Index Array(array=w484, index=w485) -> (element=w481:bool)
            n194 = Equal To 0?(x=w483) -> (x = 0?=w480:bool)
            n195 = Equal To 0?(x=w482) -> (x = 0?=w479:bool)
            n196 = Compound Arithmetic op=AND ("复合运算")(w481, w480, w479) -> (w478:bool)
          }
          frame "间隔启动" {
            n197 = Increment(x=w496) -> (x+1=w489:u32)
            n198 = Multiply(x=w494, y=u32 120) -> (x*y=w488:u32)
            n199 = Less?(x=w488, y=w489) -> (x < y?=w492:bool)
            n200 = Select(t=u32 0 ("y"), s=w492, f=w489) -> (s? t:f=w490:u32)
            n201 = Equal To 0?(x=w496) -> (x = 0?=w495:bool)
          }
        }
        n202 = call <vilib>:"Boolean Crossing PtByPt.vi"("direction"=enum16{"either", "false-true", "true-false"}."false-true", "input"=w464) -> ("crossing"=w463:bool)  [unwired: 1 in]
        n203 = case shown="True" w463 {
          tunnel: w465 -> [_ w473]
          frame False {
          }
          frame True {
            n204 = global read "断电保存变量.vi" "运行周期"() -> (w474:T14)
            n205 = Unbundle By Name(w474) -> ("运行模式"=w475:enum16{"维护模式", "常规模式", "应急模式", "质控模式"})
            n206 = case shown="\"常规模式\", Default" w475 {
              tunnel: ["M" ("数据标记表") "N" ("数据标记表")] -> w472
              frame "维护模式" {
              }
              frame "常规模式", Default {
              }
            }
            n207 = Enqueue Element(queue=w473, element=w472) -> ()  [unwired: 2 in, 3 out]
          }
        }
      }
    }
    n208 = local write "周期设置"(w453) -> ()
  }
  n209 = property class="VI"(reference=w22) -> ("Library.Version"=w21:T15)  [unwired: 1 in, 2 out]
  n210 = Equal?(x="编号", y="") -> (x = y?=w13:bool)
  n211 = Select(t="1", s=w13, f="编号") -> (s? t:f=w11:string)
  n212 = Unbundle By Name(w21) -> ("Major"=w19:u16, "Minor"=w18:u16, "Fix"=w17:u16, "Build"=w16:u16)
  n213 = global write "多参数全局变量.vi" "多参数编号"(w11) -> ()
  n214 = call "配置读取.vi"() -> ("error out"=w2:errorcluster)  [unwired: 11 in]
  n215 = Format Into String(format string="模块版本号：%d.%d.%d.%d" ("格式字符串"), w19, w18, w17, w16) -> (resulting string=→"模块版本号":string)  [unwired: 2 in, 1 out]
  n216 = case shown="\"假\", Default" w11 {
    tunnel: [TRUE ("可见") FALSE ("可见")] -> w23
    frame "假", Default {
    }
    frame "001" {
    }
  }
  n217 = Concatenate Strings("MPresource" ("名称（未命名）"), w11) -> (w29:string)
  n218 = call <vilib>:"Clear Errors.vi"("error in (no error)"=w2) -> ("error out"=w1:errorcluster)  [unwired: 5 in, 1 out]
  n219 = Concatenate Strings("MPP" ("名称（未命名）"), w11) -> (w30:string)
  n220 = Obtain Queue(name (unnamed)=w29, element data type="" ("名称（未命名）")) -> (queue out=w26:refnum<queue>)  [unwired: 3 in, 2 out]
  n221 = property on="窗格" class="Pane"("Origin"=T5 {"Horizontal"=0, "Vertical"=0} ("原点")) -> (error out=w36:errorcluster)  [unwired: 2 in, 1 out]
  n222 = Obtain Queue(name (unnamed)="MT NET Write" ("名称（未命名）"), element data type=T4 {"cmd"=enum."水样测试", "data"=variant} ("簇")) -> (queue out=w7:refnum<queue>)  [unwired: 3 in, 2 out]
  n223 = Obtain Notifier(name (unnamed)=w30, notification data type=FALSE, error in (no error)=w1) -> (notifier out=w6:refnum<notifier>, error out=w3:errorcluster)  [unwired: 1 in, 1 out]
  n224 = Enqueue Element(queue=w26, element="open" ("元素")) -> (queue out=w25:refnum<queue>)  [unwired: 2 in, 2 out]
  n225 = while {
    tunnel: w25 -> [w500]
    stop <- FALSE stop-if-true
    # "断线重连"
    n226 = Wait (ms)(milliseconds to wait=u32 10000 ("等待时间（毫秒）")) -> ()  [unwired: 1 out]
    n227 = global read "断电保存变量.vi" "连接方式"() -> (w501:u16)
    n228 = case shown="1" w501 {
      tunnel: w500 -> [_ w504]
      frame 0, Default {
      }
      frame 1 {
        n229 = case shown="True" "自动断线重连" {
          tunnel: w504 -> [_ w507]
          frame False {
          }
          frame True {
            n230 = global read "多参数全局变量.vi" "MB session in"() -> (w506:refnum<class "MB_Master.lvclass">)
            n231 = property class="MB_Master"(reference=w506) -> ("Properties:Session Valid"=w505:bool)  [unwired: 1 in, 2 out]
            n232 = case shown="False" w505 {
              tunnel: w507 -> [w508 _]
              frame False {
                n233 = Flush Queue(queue=w508) -> (queue out=w510:refnum<queue>)  [unwired: 1 in, 2 out]
                n234 = Enqueue Element(queue=w510, element="open" ("元素")) -> ()  [unwired: 2 in, 3 out]
              }
              frame True {
              }
            }
          }
        }
      }
    }
  }
  n235 = property on="编号" class="Str"("Visible"=w23) -> ()  [unwired: 2 in, 2 out]
  n236 = call "多参数 interface.vi"("error in (no error)"=w3) -> ()  [unwired: 11 in]
  n237 = call "taskqueue ref.vi"() -> ("队列输出"=w4:refnum<queue>)  [unwired: 10 in, 1 out]
  n238 = flat-sequence {
    tunnel: w3 -> [_]
    frame #0 {
      n239 = local read "编号"() -> (w512:string)
      n240 = Equal?(x=w512, y="") -> (x = y?=w514:bool)
      n241 = Select(t="1", s=w514, f=w512) -> (s? t:f=w511:string)
      n242 = call "探头数据读取.vi"("编号"=w511) -> ()  [unwired: 11 in]
    }
  }
  n243 = while {
    tunnel: w25 -> [w517]
    tunnel: w3 -> [_]
    stop <- FALSE stop-if-true
    n244 = Dequeue Element(queue=w517) -> (element=w516:string)  [unwired: 2 in, 3 out]
    n245 = case shown="\"open\"" w516 {
      tunnel: [_ w520 w529] -> _
      frame "假", Default {
      }
      frame "open" {
        n246 = global read "多参数全局变量.vi" "MB session in"() -> (w525:refnum<class "MB_Master.lvclass">)
        n247 = global read "断电保存变量.vi" "VISA资源名称"() -> (w526:refnum<visa-resource-name>)
        n248 = global read "断电保存变量.vi" "Serial Config"() -> (w519:T1)
        n249 = global read "断电保存变量.vi" "连接方式"() -> (w523:u16)
        n250 = call "close MB.vi"("MB session in"=w525) -> ("error out"=w527:errorcluster)  [unwired: 10 in]
        n251 = global read "断电保存变量.vi" "Port"() -> (w521:u16)
        n252 = global read "断电保存变量.vi" "IP"() -> (w522:string)
        n253 = call "open MB.vi"("Port (502)"=w521, "IP Address"=w522, "MODE"=w523, "error in (no error)"=w527, "Serial Config"=w519, "VISA资源名称"=w526) -> ("error out"=w520:errorcluster, "MB session out"=w524:refnum<class "MB_Master.lvclass">)  [unwired: 4 in]
        n254 = global write "多参数全局变量.vi" "MB session in"(w524) -> ()
      }
      frame "close" {
        n255 = global read "多参数全局变量.vi" "MB session in"() -> (w528:refnum<class "MB_Master.lvclass">)
        n256 = call "close MB.vi"("MB session in"=w528) -> ("error out"=w529:errorcluster)  [unwired: 10 in]
      }
    }
  }
  n257 = while {
    tunnel: [w539] -> _
    shift-right: [w533] -> _
    shift-left: _ -> [w537]
    tunnel: w3 -> [w534]
    stop <- FALSE stop-if-true
    n258 = Wait (ms)(milliseconds to wait=u32 1000 ("等待时间（毫秒）")) -> ()  [unwired: 1 out]
    n259 = call <vilib>:"Application Directory.vi"() -> ("Application Directory"=w532:path)
    n260 = Build Path(base path=w532, name or relative path="data\\DCSset.ini" ("名称或相对路径")) -> (appended path=w530:path)
    n261 = File/Directory Info(path=w530, error in=w534) -> (last mod=w533:timestamp, error out=w535:errorcluster)  [unwired: 5 out]
    n262 = Not Equal?(x=w533, y=w537) -> (x != y?=w536:bool)
    n263 = case shown="True" w536 {
      tunnel: [w541 w549] -> w539
      tunnel: w535 -> [w541 w548]
      tunnel: w530 -> [_ w542]
      frame False {
      }
      frame True {
        # "文件发生改变进行更新"
        n264 = call <vilib>:"Open Config Data.vi"("error in (no error)"=w548, "configuration file path"=w542) -> ("error out"=w547:errorcluster, "refnum"=w546:T16)  [unwired: 7 in, 1 out]
        n265 = vi-ref "断电保存变量.vi"() -> (w543:refnum<vi>)
        n266 = call <userlib>:"Read Panel from INI__ogtk.vi"("error in (no error)"=w547, "VI ref"=w543, "refnum"=w546) -> ("error out"=w545:errorcluster, "refnum out"=w544:T16)  [unwired: 7 in]
        n267 = call <vilib>:"Close Config Data.vi"("error in (no error)"=w545, "refnum"=w544) -> ("error out"=w549:errorcluster)  [unwired: 8 in, 1 out]
      }
    }
  }
  n268 = flat-sequence {
    tunnel: w6 -> [w551]
    frame #0 {
      n269 = Obtain Queue(name (unnamed)="MT NET Read" ("名称（未命名）"), element data type=T4 {"cmd"=enum."水样测试", "data"=variant} ("簇")) -> (queue out=w553:refnum<queue>)  [unwired: 3 in, 2 out]
      n270 = call "taskqueue ref.vi"() -> ("队列输出"=w550:refnum<queue>)  [unwired: 10 in, 1 out]
      n271 = while {
        tunnel: w553 -> [w560]
        tunnel: [w558] -> w554
        tunnel: w551 -> [w557]
        tunnel: w550 -> [w556]
        stop <- FALSE stop-if-true
        n272 = Dequeue Element(queue=w560) -> (queue out=w558:refnum<queue>, element=w559:T4)  [unwired: 2 in, 2 out]
        n273 = flat-sequence {
          tunnel: w559 -> [w566]
          tunnel: w557 -> [w563]
          tunnel: w556 -> [w562]
          frame #0 {
            n274 = Unbundle By Name(w566) -> ("cmd"=w565:enum16{"水样测试", "标样核查", "校准状态同步", "停止"}, "data"=w564:variant)
            n275 = case shown="\"标样核查\"" w565 {
              tunnel: w564 -> [w569 _ _ w596]
              tunnel: w563 -> [_ _ w592 _]
              tunnel: w562 -> [w568 _ _ _]
              frame "水样测试", Default {
                n276 = Get Queue Status(queue=w568) -> (# elements in queue=w567:i32)  [unwired: 2 in, 7 out]
                n277 = case shown="0" w567 {
                  tunnel: w569 -> [_ w574]
                  tunnel: w568 -> [_ w571]
                  frame Default {
                  }
                  frame 0 {
                    n278 = global read "断电保存变量.vi" "运行周期"() -> (w576:T14)
                    n279 = Unbundle By Name(w576) -> ("运行模式"=w575:enum16{"维护模式", "常规模式", "应急模式", "质控模式"})
                    n280 = Variant To Data(type="", Variant=w574) -> (data=w572:string)  [unwired: 1 in, 1 out]
                    n281 = case shown="\"常规模式\", Default" w575 {
                      tunnel: ["M" ("数据标记表") w579] -> w570
                      tunnel: w572 -> [_ w578]
                      frame "维护模式" {
                      }
                      frame "常规模式", Default {
                        n282 = case shown="Default" w578 {
                          selector: w578 -> [_ w581]
                          tunnel: ["N" ("数据标记表") w581] -> w579
                          frame Default {
                          }
                          frame "hd" {
                          }
                        }
                      }
                    }
                    n283 = Enqueue Element(queue=w571, element=w570) -> ()  [unwired: 2 in, 3 out]
                  }
                }
              }
              frame "标样核查" {
                n284 = vi-ref "标样核查.vi"() -> (w583:refnum<vi>)
                n285 = property class="VI"(reference=w583) -> ("Name"=w587:string, "Exec.State"=w585:T17)  [unwired: 1 in, 2 out]
                n286 = Open VI Reference(type specifier VI Refnum (for type only)=refnum<vi> refnum, vi path=w587, options=128 ("选项")) -> (vi reference=w588:refnum<vi>)  [unwired: 3 in, 1 out]
                n287 = case shown="\"Idle\"" w585 {
                  tunnel: [w589 w591] -> w584
                  tunnel: w588 -> [w589 w590]
                  frame "Bad", Default {
                  }
                  frame "Idle" {
                    n288 = call-by-ref "开始异步调用"(reference=w590) -> (reference out=w591:refnum<vi>)  [unwired: 13 in, 1 out]
                  }
                }
                n289 = Close Reference(reference=w584) -> ()  [unwired: 1 in, 1 out]
              }
              frame "停止" {
                n290 = Send Notification(notification=TRUE ("通知"), notifier=w592) -> ()  [unwired: 1 in, 2 out]
              }
              frame "校准状态同步" {
                n291 = global read "多参数全局变量.vi" "远程校准运行状态"() -> (w595:T18)
                n292 = Variant To Data(type=w595, Variant=w596) -> (data=w594:T18)  [unwired: 1 in, 1 out]
                n293 = global write "多参数全局变量.vi" "远程校准运行状态"(w594) -> ()
              }
            }
          }
        }
      }
      n294 = call "数据流读取.vi"() -> ()  [unwired: 12 in]
      n295 = call "数据流写入.vi"() -> ()  [unwired: 12 in]
      n296 = Release Queue(queue=w554) -> ()  [unwired: 2 in, 3 out]
    }
  }
  n297 = while {
    tunnel: w36 -> [_]
    tunnel: w6 -> [w600]
    tunnel: w25 -> [w599]
    tunnel: w7 -> [w598]
    tunnel: w4 -> [w597]
    stop <- FALSE stop-if-true
    n298 = event shown="[18] \"探头校正\": Value Change" {
      selector: _ -> [_ _ _ _ _ _ _ _ _ _ _ _ _ _ _ _ _ _ _]
      dyn-events: _ -> [_ _ _ _ _ _ _ _ _ _ _ _ _ _ _ _ _ _ _]
      timeout: _ -> [_ _ _ _ _ _ _ _ _ _ _ _ _ _ _ _ _ _ _]
      tunnel: w600 -> [_ _ _ _ _ _ _ _ _ _ _ _ _ w670 _ _ _ _ _]
      tunnel: w599 -> [_ _ _ _ _ _ _ _ _ _ _ _ _ _ _ _ w682 _ _]
      tunnel: w598 -> [_ _ _ _ _ _ _ _ _ _ _ w645 w653 w668 _ _ _ _ _]
      tunnel: w597 -> [_ _ _ _ _ _ _ _ _ _ _ w641 _ _ _ _ _ _ _]
      event Timeout {
        n299 = event-data() -> ()  [unwired: 1 in, 3 out]
      }
      event "探头设置": Value Change {
        n300 = event-data() -> ()  [unwired: 1 in, 6 out]
        n301 = call "探头启用设置.vi"() -> ()  [unwired: 12 in]
      }
      event "量程设置": Value Change {
        n302 = event-data() -> ()  [unwired: 1 in, 6 out]
        n303 = global read "断电保存变量.vi" "量程参数"() -> (w604:T19)
        n304 = call "量程参数设置对话框.vi"("量程参数"=w604) -> ("布尔"=w602:bool, "量程参数 2"=w603:T19)  [unwired: 9 in]
        n305 = case shown="True" w602 {
          tunnel: w603 -> [_ w605]
          frame False {
          }
          frame True {
            n306 = flat-sequence {
              tunnel: w605 -> [w606]
              frame #0 {
                n307 = global write "断电保存变量.vi" "量程参数"(w606) -> ()
              }
              frame #1 {
                n308 = call "配置文件保存.vi"() -> ()  [unwired: 12 in]
              }
            }
          }
        }
      }
      event "传感器系列号": Value Change {
        n309 = event-data() -> ()  [unwired: 1 in, 6 out]
        n310 = call "系列号查询.vi"() -> ()  [unwired: 12 in]
      }
      event "水样稳定时间", "水样保存组数": Mouse Down {
        n311 = event-data() -> ("CtlRef"=w607:refnum<vi>)  [unwired: 1 in, 7 out]
        n312 = property class="DigNum (strict)"(reference=w607) -> (reference out=w610:refnum<vi>, "Value"=w609:dbl)  [unwired: 1 in, 1 out]
        n313 = call "数字键盘.vi"("OldNumber"=w609) -> ("NewNumber"=w608:dbl)  [unwired: 1 in]
        n314 = property class="DigNum (strict)"(reference=w610, "Val(Sgnl)"=w608) -> ()  [unwired: 1 in, 2 out]
      }
      event "VISA资源名称", "打开modbus", "连接方式", "自动断线重连": Mouse Down {
        n315 = event-data() -> ()  [unwired: 1 in, 6 out]
        n316 = local read "密码锁"() -> (w611:bool)
        n317 = case shown="False" w611 {
          frame False {
            n318 = One Button Dialog(message="当前操作权限不足,请提升权限!!!" ("消息")) -> ()  [unwired: 1 in, 1 out]
          }
          frame True {
          }
        }
      }
      event "IP": Mouse Down {
        n319 = event-data() -> ("CtlRef"=w614:refnum<vi>)  [unwired: 1 in, 7 out]
        n320 = property on="IP" class="Str"() -> ("DisabledEnum"=w613:T6)  [unwired: 2 in, 2 out]
        n321 = case shown="\"Disabled and Grayed Out\"" w613 {
          tunnel: w614 -> [w618 _ _]
          frame "Enabled" {
            n322 = property class="Str"(reference=w618) -> (reference out=w617:refnum<vi>, "Value"=w616:string)  [unwired: 1 in, 1 out]
            n323 = call "字符键盘.vi"("Old String"=w616) -> ("String"=w615:string)  [unwired: 10 in]
            n324 = property class="Str"(reference=w617, "Val(Sgnl)"=w615) -> ()  [unwired: 1 in, 2 out]
          }
          frame "Disabled and Grayed Out" {
            n325 = One Button Dialog(message="关闭连接后才可设置!" ("消息")) -> ()  [unwired: 1 in, 1 out]
          }
          frame "Disabled", Default {
            n326 = One Button Dialog(message="当前操作权限不足,请提升权限!!!" ("消息")) -> ()  [unwired: 1 in, 1 out]
          }
        }
      }
      event "Port": Mouse Down {
        n327 = event-data() -> ("CtlRef"=w622:refnum<vi>)  [unwired: 1 in, 7 out]
        n328 = property on="Port" class="DigNum (strict)"() -> ("DisabledEnum"=w621:T6)  [unwired: 2 in, 2 out]
        n329 = case shown="\"Enabled\"" w621 {
          tunnel: w622 -> [w626 _ _]
          frame "Enabled" {
            n330 = property class="DigNum (strict)"(reference=w626) -> (reference out=w625:refnum<vi>, "Value"=w624:u16)  [unwired: 1 in, 1 out]
            n331 = call "数字键盘.vi"("OldNumber"=w624) -> ("NewNumber"=w623:dbl)  [unwired: 1 in]
            n332 = property class="DigNum (strict)"(reference=w625, "Val(Sgnl)"=w623) -> ()  [unwired: 1 in, 2 out]
          }
          frame "Disabled and Grayed Out" {
            n333 = One Button Dialog(message="关闭连接后才可设置!" ("消息")) -> ()  [unwired: 1 in, 1 out]
          }
          frame "Disabled", Default {
            n334 = One Button Dialog(message="当前操作权限不足,请提升权限!!!" ("消息")) -> ()  [unwired: 1 in, 1 out]
          }
        }
      }
      event "密码锁": Value Change {
        n335 = event-data() -> ("NewVal"=w629:bool)  [unwired: 1 in, 5 out]
        n336 = case shown="True" w629 {
          frame False {
            n337 = global write "多参数全局变量.vi" "权限"(enum16{"一级权限", "二级权限", "三级权限"}."一级权限" ("权限")) -> ()
          }
          frame True {
            n338 = global read "多参数全局变量.vi" "权限密码"() -> (w632:u32[])
            n339 = global read "多参数全局变量.vi" "权限"() -> (w631:enum16{"一级权限", "二级权限", "三级权限", "超级权限"})
            n340 = call "密码权限设置.vi"("权限输入"=w631, "权限密码"=w632) -> ("权限"=w633:enum16{"一级权限", "二级权限", "三级权限", "超级权限"})  [unwired: 9 in]
            n341 = global write "多参数全局变量.vi" "权限"(w633) -> ()
          }
        }
      }
      event "权限等级": Mouse Down {
        n342 = event-data() -> ()  [unwired: 1 in, 8 out]
        n343 = global read "多参数全局变量.vi" "权限密码"() -> (w636:u32[])
        n344 = global read "多参数全局变量.vi" "权限"() -> (w634:enum16{"一级权限", "二级权限", "三级权限", "超级权限"})
        n345 = call "密码权限设置.vi"("权限输入"=w634, "权限密码"=w636) -> ("权限"=w635:enum16{"一级权限", "二级权限", "三级权限", "超级权限"})  [unwired: 9 in]
        n346 = global write "多参数全局变量.vi" "权限"(w635) -> ()
      }
      event "周期设置": Mouse Down {
        n347 = event-data() -> ()  [unwired: 1 in, 6 out]
        n348 = flat-sequence {
          frame #0 {
            n349 = global read "断电保存变量.vi" "定时控制输入"() -> (w638:T12)
            n350 = call "周期设置.vi"("定时控制输入"=w638) -> ("定时控制输出"=w637:T20)  [unwired: 10 in]
            n351 = global write "断电保存变量.vi" "定时控制输入"(w637) -> ()
          }
          frame #1 {
            n352 = call "配置文件保存.vi"() -> ()  [unwired: 12 in]
          }
        }
      }
      event "水样测试": Value Change {
        n353 = event-data() -> ()  [unwired: 1 in, 6 out]
        n354 = Get Queue Status(queue=w641) -> (queue out=w639:refnum<queue>, # elements in queue=w640:i32)  [unwired: 2 in, 6 out]
        n355 = case shown="0" w640 {
          tunnel: w639 -> [_ w647]
          frame Default {
          }
          frame 0 {
            n356 = global read "断电保存变量.vi" "运行周期"() -> (w650:T14)
            n357 = Unbundle By Name(w650) -> ("运行模式"=w649:enum16{"维护模式", "常规模式", "应急模式", "质控模式"})
            n358 = case shown="\"常规模式\", Default" w649 {
              tunnel: ["M" ("数据标记表") w652] -> w646
              tunnel: "hd" ("数据标记表") -> [_ w652]
              frame "维护模式" {
              }
              frame "常规模式", Default {
              }
            }
            n359 = Enqueue Element(queue=w647, element=w646) -> ()  [unwired: 2 in, 3 out]
          }
        }
        n360 = Bundle By Name(cluster=T4 {"cmd"=enum."水样测试", "data"=variant} ("元素"), "data"="hd" ("数据标记表")) -> (w642:T4)
        n361 = Enqueue Element(queue=w645, element=w642) -> ()  [unwired: 2 in, 3 out]
      }
      event "标样核查": Value Change {
        n362 = event-data() -> ()  [unwired: 1 in, 6 out]
        n363 = call "标样核查配置.vi"() -> ("确认输出"=w654:bool)  [unwired: 11 in]
        n364 = case shown="True" w654 {
          tunnel: w653 -> [_ w663]
          frame False {
          }
          frame True {
            n365 = vi-ref "标样核查.vi"() -> (w656:refnum<vi>)
            n366 = property class="VI"(reference=w656) -> ("Name"=w660:string, "Exec.State"=w658:T17)  [unwired: 1 in, 2 out]
            n367 = Enqueue Element(queue=w663, element=T4 {"cmd"=enum."标样核查", "data"=variant} ("元素")) -> ()  [unwired: 2 in, 3 out]
            n368 = Open VI Reference(type specifier VI Refnum (for type only)=refnum<vi> refnum, vi path=w660, options=128 ("选项")) -> (vi reference=w661:refnum<vi>)  [unwired: 3 in, 1 out]
            n369 = case shown="\"Idle\"" w658 {
              tunnel: [w664 w666] -> w657
              tunnel: w661 -> [w664 w665]
              frame "Bad", Default {
              }
              frame "Idle" {
                n370 = call-by-ref "开始异步调用"(reference=w665) -> (reference out=w666:refnum<vi>)  [unwired: 13 in, 1 out]
              }
            }
            n371 = Close Reference(reference=w657) -> ()  [unwired: 1 in, 1 out]
          }
        }
      }
      event "停止": Value Change {
        n372 = event-data() -> ()  [unwired: 1 in, 6 out]
        n373 = Send Notification(notification=TRUE ("通知"), notifier=w670) -> ()  [unwired: 1 in, 2 out]
        n374 = Enqueue Element(queue=w668, element=T4 {"cmd"=enum."停止", "data"=variant} ("元素")) -> ()  [unwired: 2 in, 3 out]
      }
      event "设置": Value Change {
        n375 = event-data() -> ()  [unwired: 1 in, 6 out]
        n376 = property on="窗格" class="Pane"("Origin"=T5 {"Horizontal"=0, "Vertical"=628} ("原点")) -> ()  [unwired: 2 in, 2 out]
        n377 = global write "多参数全局变量.vi" "当前页面"(enum16{"主页面", "参数页面", "校准页面"}."参数页面" ("当前页面")) -> ()
      }
      event "VISA资源名称", "连接方式", "IP", "Port", "自动断线重连", "水样稳定时间", "水样保存组数", "Serial Config": Value Change {
        n378 = event-data() -> ()  [unwired: 1 in, 6 out]
        n379 = flat-sequence {
          frame #0 {
            n380 = global write "断电保存变量.vi" "IP"("IP") -> ()
            n381 = global write "断电保存变量.vi" "Port"("Port") -> ()
            n382 = global write "断电保存变量.vi" "连接方式"("连接方式") -> ()
            n383 = local read "自动断线重连"() -> (w676:bool)
            n384 = global write "断电保存变量.vi" "Serial Config"("Serial Config") -> ()
            n385 = global write "断电保存变量.vi" "水样测试组数"("水样保存组数") -> ()
            n386 = global write "断电保存变量.vi" "水样稳定时间"("水样稳定时间") -> ()
            n387 = global write "断电保存变量.vi" "VISA资源名称"("VISA资源名称") -> ()
            n388 = global write "断电保存变量.vi" "自动断线重连"(w676) -> ()
          }
          frame #1 {
            n389 = call "配置文件保存.vi"() -> ()  [unwired: 12 in]
          }
          frame #2 {
          }
        }
      }
      event "打开modbus": Value Change {
        n390 = event-data() -> ()  [unwired: 1 in, 6 out]
        n391 = global read "多参数全局变量.vi" "MB session in"() -> (w687:refnum<class "MB_Master.lvclass">)
        n392 = Flush Queue(queue=w682) -> (queue out=w681:refnum<queue>)  [unwired: 1 in, 2 out]
        n393 = property class="MB_Master"(reference=w687) -> ("Properties:Session Valid"=w686:bool)  [unwired: 1 in, 2 out]
        n394 = Select(t="close" ("元素"), s=w686, f="open" ("元素")) -> (s? t:f=w683:string)
        n395 = Enqueue Element(queue=w681, element=w683) -> ()  [unwired: 2 in, 3 out]
      }
      event "探头校正返回", "设置页返回": Value Change {
        n396 = event-data() -> ()  [unwired: 1 in, 6 out]
        n397 = property on="窗格" class="Pane"("Origin"=T5 {"Horizontal"=0, "Vertical"=0} ("原点")) -> ()  [unwired: 2 in, 2 out]
        n398 = global write "多参数全局变量.vi" "当前页面"(enum16{"主页面", "参数页面", "校准页面"}."主页面" ("当前页面")) -> ()
      }
      event "探头校正": Value Change {
        n399 = event-data() -> ()  [unwired: 1 in, 6 out]
        n400 = global write "多参数全局变量.vi" "当前页面"(enum16{"主页面", "参数页面", "校准页面"}."校准页面" ("当前页面")) -> ()
        n401 = property on="窗格" class="Pane"("Origin"=T5 {"Horizontal"=1656, "Vertical"=0} ("原点")) -> ()  [unwired: 2 in, 2 out]
        n402 = vi-ref "斯坦道多参数.lvlib:校准Main.vi"() -> (w691:refnum<vi>)
        n403 = property class="VI"(reference=w691) -> (reference out=w693:refnum<vi>, "Exec.State"=w692:T17)  [unwired: 1 in, 1 out]
        n404 = case shown="\"Bad\", Default" w692 {
          tunnel: [w697 w699] -> w695
          tunnel: w693 -> [w697 w698]
          frame "Bad", Default {
          }
          frame "Idle" {
            n405 = invoke class="VI" method="Run VI"(reference=w698, "Wait until done"=FALSE ("结束前等待"), "Auto Dispose Ref"=FALSE ("自动销毁引用")) -> (reference out=w699:refnum<vi>)  [unwired: 2 in, 4 out]
          }
        }
        n406 = invoke on="探头校准子面板" class="SubPnl" method="Remove VI"() -> (error out=w694:errorcluster)  [unwired: 3 in, 2 out]
        n407 = invoke on="探头校准子面板" class="SubPnl" method="Insert VI"(error in=w694, "VI Ref"=w695) -> ()  [unwired: 2 in, 4 out]
      }
    }
  }
